vi "applyDelaysToDevice.vi"(8 "error in (no error)":errorcluster, 10 "device":refnum<class "device.lvclass">, 11 "ScriptListCompiler in":refnum<class "ScriptListCompiler.lvclass">) -> (0 "error out":errorcluster, 2 "device out":refnum<class "device.lvclass">, 3 "ScriptListCompiler out":refnum<class "ScriptListCompiler.lvclass">)   [LabVIEW 2011, in "Compiler.lvlib" / "ScriptListCompiler.lvclass"]
uses:
  ScriptListCompiler.lvclass
  DatabaseHelpers/Database Objects/device/device.lvclass
  Scripting/ScriptingEvent/ScriptEventList/ScriptEventList.lvclass
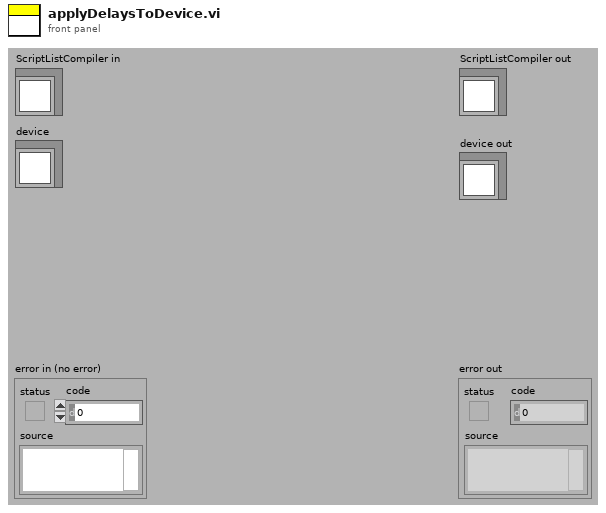
[diagram p1: front panel]
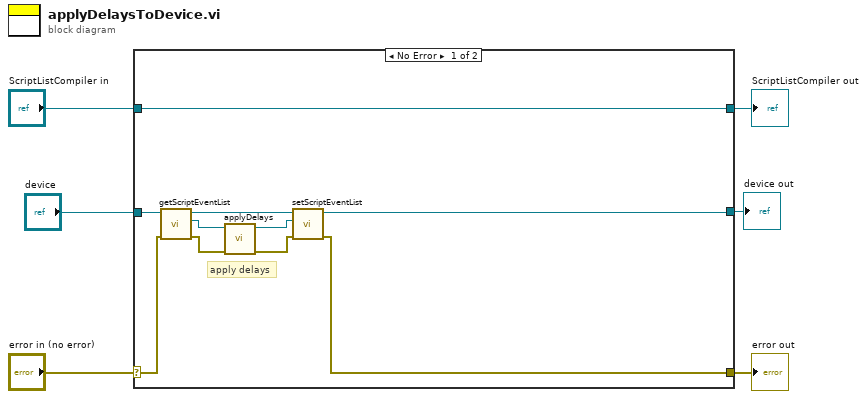
[diagram p0: block diagram]
diagram:
  n1 = case shown="No Error" "error in (no error)" {
    selector: "error in (no error)" -> [w14 w18]
    tunnel: [w8 w18] -> w5
    tunnel: [w16 w17] -> w3
    tunnel: "ScriptListCompiler in" -> [w16 w17]
    tunnel: "device" -> [w15 _]
    tunnel: [w7 _] -> w1
    frame No Error {
      # "apply delays"
      n2 = call "getScriptEventList.vi"("error in (no error)"=w14, "device.lvclass in"=w15) -> ("error out"=w12:errorcluster, "ScriptEventList"=w13:refnum<class "ScriptEventList.lvclass">, "device.lvclass out"=w11:refnum<class "device.lvclass">)  [unwired: 7 in]
      n3 = call "applyDelays.vi"("error in (no error)"=w12, "ScriptEventList in"=w13) -> ("error out"=w9:errorcluster, "ScriptEventList out"=w10:refnum<class "ScriptEventList.lvclass">)  [unwired: 8 in]
      n4 = call "setScriptEventList.vi"("error in (no error)"=w9, "ScriptEventList"=w10, "device.lvclass in"=w11) -> ("error out"=w8:errorcluster, "device.lvclass out"=w7:refnum<class "device.lvclass">)  [unwired: 7 in]
    }
    frame Error {
    }
  }
  "error out" <- w5
  "ScriptListCompiler out" <- w3
  "device out" <- w1
